vi "Start.vi"(8 "error in (no error)":errorcluster, 10 "Params":variant, 11 "AnalysisPluginsBase in":refnum<class "AnalysisPluginsBase.lvclass">) -> (0 "error out":errorcluster, 3 "AnalysisPluginsBase out":refnum<class "AnalysisPluginsBase.lvclass">)   [LabVIEW 2018, in "AnalysisPlugins.lvlib" / "AnalysisPluginsBase.lvclass"]
uses:
  AnalysisPluginsBase.lvclass
  Typedefs/SampleDataInput.ctl
  Typedefs/clWindowData.ctl
  AnalysisPluginsBase.lvclass/AnalysisPluginsBase.ctl
  Accessors/Read SampleDataQueName.vi
  Accessors/Write SampleDataInput.vi
  Accessors/Write Window.vi
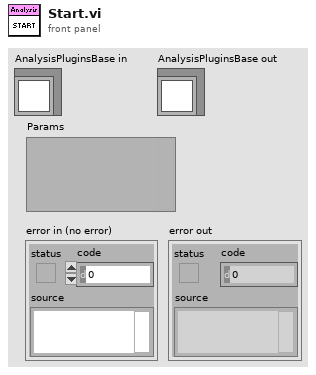
[diagram p1: front panel]
types:
  T1 = typedef "AnalysisPlugins.lvlib/AnalysisPluginsBase.lvclass/clWindowData.ctl" = cluster{"Timestamp":ext, "Samples":dbl[][], "Window Valid":bool, "T0":ext}
  T2 = typedef "AnalysisPlugins.lvlib/AnalysisPluginsBase.lvclass/SampleDataInput.ctl" = waveform(dbl)[]
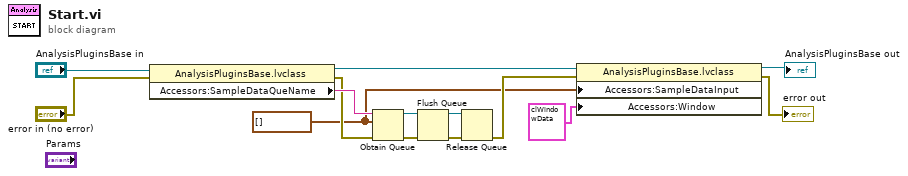
[diagram p0: block diagram]
diagram:
  w4 = T2 [] ("clSampleDataArray")
  n1 = property class="AnalysisPluginsBase.lvclass"(reference="AnalysisPluginsBase in", error in="error in (no error)") -> (reference out=w6:refnum<class "AnalysisPluginsBase.lvclass">, error out=w11:errorcluster, "Accessors:SampleDataQueName"=w12:string)
  n2 = Obtain Queue(name (unnamed)=w12, element data type=w4, error in (no error)=w11) -> (queue out=w9:refnum<queue>, error out=w10:errorcluster)  [unwired: 2 in, 1 out]
  n3 = Flush Queue(queue=w9, error in (no error)=w10) -> (queue out=w7:refnum<queue>, error out=w8:errorcluster)  [unwired: 1 out]
  n4 = Release Queue(queue=w7, error in (no error)=w8) -> (error out=w5:errorcluster)  [unwired: 1 in, 2 out]
  n5 = property class="AnalysisPluginsBase.lvclass"(reference=w6, error in=w5, "Accessors:SampleDataInput"=w4, "Accessors:Window"=T1 {"Timestamp"=0.0, "Samples"=[], "Window Valid"=FALSE, "T0"=0.0} ("Window")) -> (reference out=→"AnalysisPluginsBase out":refnum<class "AnalysisPluginsBase.lvclass">, error out=→"error out":errorcluster)
